vi "Splash VI Path.vi"() -> (2 "Splash VI Path":path)   [LabVIEW 2020, in "Volatus.lvlib" / "Plugin Splash.lvclass"]
uses:
  Plugin Splash.lvclass
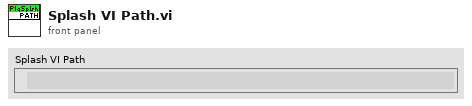
[diagram p1: front panel]
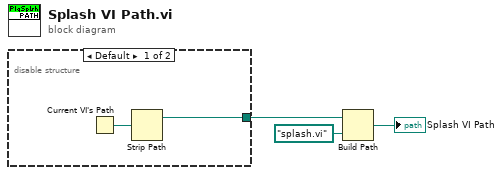
[diagram p0: block diagram]
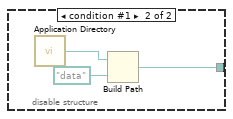
[diagram p2: hidden frame]
diagram:
  n1 = disable-structure shown="Default" {
    disable-tunnel: [w4 w6] -> w3
    frame condition #0 (active) {
      n2 = Current VI's Path() -> (path=w5:path)
      n3 = Strip Path(path=w5) -> (stripped path=w4:path)  [unwired: 1 out]
    }
    frame condition #1 {
      n4 = call <vilib>:"Application Directory.vi"() -> ("Application Directory"=w8:path)
      n5 = Build Path(base path=w8, name or relative path=path "data") -> (appended path=w6:path)
    }
  }
  n6 = Build Path(base path=w3, name or relative path=path "splash.vi") -> (appended path=→"Splash VI Path":path)
